vi "Init_Data_Core.vi"(8 "error in":errorcluster, 11 "Subpanel":refnum<vi>) -> (0 "error out":errorcluster, 3 "Data Out":T1)   [LabVIEW 2020]
uses:
  Type Defs/Data_Core.ctl
  src/vectorstore/vector_qdrant/vector_qdrant.lvclass
  src/models/llm_openai_chatmodels/llm_openai_chatmodels.lvclass
  src/models/llm_openai_embedding/llm_openai_embedding.lvclass
  src/user_interfaces/simple_html_chat_ui/simple_html_chat_ui.lvclass
  src/models/llm_openai_embedding/Instantiate_llm_openai_embed.vi
  src/models/llm_openai_chatmodels/Instantiate_llm_openai.vi
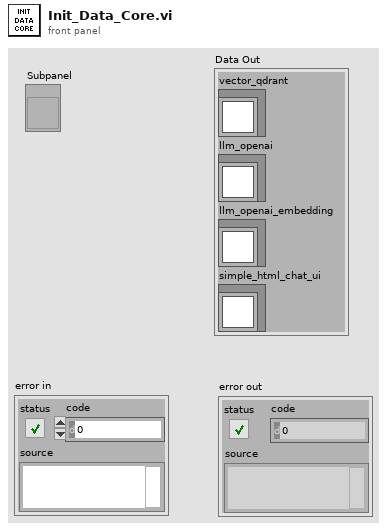
[diagram p1: front panel]
types:
  T1 = typedef "Data_Core.ctl" = cluster{"vector_qdrant":refnum<class "vector_qdrant.lvclass">, "llm_openai":refnum<class "llm_openai_chatmodels.lvclass">, "llm_openai_embedding":refnum<class "llm_openai_embedding.lvclass">, "simple_html_chat_ui":refnum<class "simple_html_chat_ui.lvclass">}
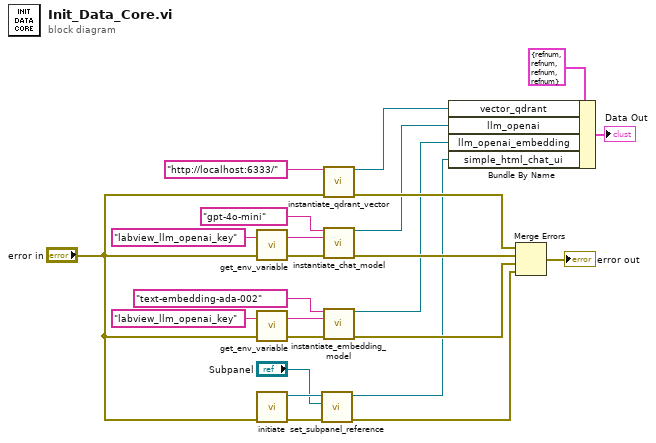
[diagram p0: block diagram]
diagram:
  n1 = call "get_env_variable.vi"("Environment Variable Name"="labview_llm_openai_key") -> ("Value"=w20:string)  [unwired: 1 in, 1 out]
  n2 = call "get_env_variable.vi"("Environment Variable Name"="labview_llm_openai_key") -> ("Value"=w16:string)  [unwired: 1 in, 1 out]
  n3 = call "initiate.vi"("error in (no error)"="error in") -> ("error out"=w15:errorcluster, "simple_html_chat_ui out"=w14:refnum<class "simple_html_chat_ui.lvclass">)  [unwired: 9 in]
  n4 = call "set_subpanel_reference.vi"("error in (no error)"=w15, "Sub Panel"="Subpanel", "simple_html_chat_ui in"=w14) -> ("error out"=w9:errorcluster, "simple_html_chat_ui out"=w5:refnum<class "simple_html_chat_ui.lvclass">)  [unwired: 7 in]
  n5 = call "instantiate_qdrant_vector.vi"("host_url"="http://localhost:6333/", "error in"="error in") -> ("vector_qdrant out"=w2:refnum<class "vector_qdrant.lvclass">, "error out"=w12:errorcluster)  [unwired: 12 in]
  n6 = call-poly "instantiate_chat_model.vi"("model_name"="gpt-4o-mini", "openai_key"=w20, "error in (no error)"="error in") -> ("llm_openai out"=w3:refnum<class "llm_openai_chatmodels.lvclass">, "error out"=w11:errorcluster)  [unwired: 11 in]
  n7 = call-poly "instantiate_embedding_model.vi"("model_name"="text-embedding-ada-002", "openai_key"=w16, "error in (no error)"="error in") -> ("llm_openai_embedding out"=w4:refnum<class "llm_openai_embedding.lvclass">, "error out"=w10:errorcluster)  [unwired: 11 in]
  n8 = Bundle By Name(cluster=T1 {"vector_qdrant"=refnum, "llm_openai"=refnum, "llm_openai_embedding"=refnum, "simple_html_chat_ui"=refnum}, "vector_qdrant"=w2, "llm_openai"=w3, "llm_openai_embedding"=w4, "simple_html_chat_ui"=w5) -> (→"Data Out":T1)
  n9 = Merge Errors(w12, w11, w10, w9) -> (→"error out":errorcluster)
